vi "MenuSelection Response.vi"(6 "Coords":T1, 8 "error in (no error)":errorcluster, 9 "Menu Name":string, 10 "Menu Tag":string, 11 "UEF Handler1 in":refnum<class "UEF Handler2.lvclass">) -> (0 "error out":errorcluster, 3 "UEF Handler1 out":refnum<class "UEF Handler2.lvclass">)   [LabVIEW 2015, in "UEF Handler2.lvclass"]
uses:
  UEF Handler2.lvclass
  <vilib>/Utility/miscctls.llb/LVPoint32TypeDef.ctl
  <vilib>/LIEF/Forms/Rectangle/Rectangle.lvclass
  <vilib>/LIEF/Image Editor Handler/Image Editor Handler.lvclass/Image Editor Handler.ctl
  UEF Handler2.lvclass/UEF Handler2.ctl
  <vilib>/LIEF/Forms/Shape/Shape.lvclass/Shape.ctl
  <vilib>/LIEF/Forms/Rectangle/Rectangle.lvclass/Rectangle.ctl
  <vilib>/LIEF/Image Editor Handler/Read PictureRef.vi
  <vilib>/LIEF/Image Editor Handler/Read Shapes.vi
  <vilib>/LIEF/Forms/Shape/Write Color.vi
  <vilib>/LIEF/Forms/Rectangle/Write Filled.vi
  <vilib>/LIEF/Forms/Shape/Shape.lvclass
  <vilib>/LIEF/Image Editor Handler/Image Editor Handler.lvclass
  <vilib>/LIEF/Forms/Link/Link.lvclass
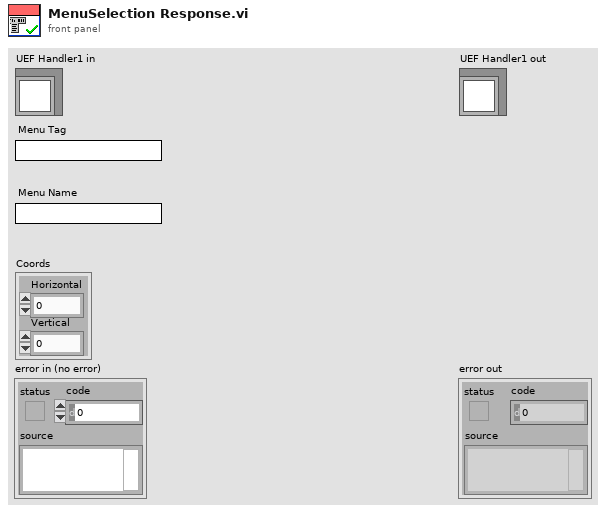
[diagram p1: front panel]
types:
  T1 = typedef "LVPoint32TypeDef.ctl" = cluster{"Horizontal":i32, "Vertical":i32}
  T2 = typedef "LVPositionTypeDef.ctl" = cluster{"Left":i32, "Top":i32}
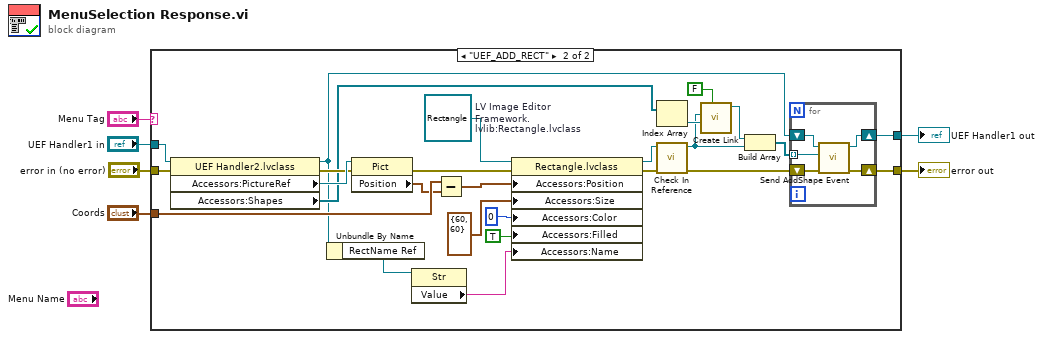
[diagram p0: block diagram]
diagram:
  n1 = case shown="\"UEF_ADD_RECT\"" "Menu Tag" {
    tunnel: "UEF Handler1 in" -> [w8 w34]
    tunnel: "Coords" -> [_ w32]
    tunnel: [w7 w23] -> w3
    tunnel: [w8 w22] -> w2
    tunnel: "error in (no error)" -> [w7 w18]
    frame "False", Default {
    }
    frame "UEF_ADD_RECT" {
      w30 = refnum<class "Rectangle.lvclass"> refnum  # LV Image Editor Framework.lvlib:Rectangle.lvclass
      n2 = property class="UEF Handler2.lvclass"(reference=w34, error in=w18) -> (reference out=w11:refnum<class "UEF Handler2.lvclass">, error out=w19:errorcluster, "Accessors:PictureRef"=w33:refnum<vi>, "Accessors:Shapes"=w17:refnum<data-value>[])
      n3 = Unbundle By Name(w11) -> ("RectName Ref"=w10:refnum<vi>)
      n4 = property class="Pict"(reference=w33, error in=w19) -> (error out=w20:errorcluster, "Position"=w31:T2)  [unwired: 1 out]
      n5 = property class="Str"(reference=w10) -> ("Value"=w9:string)  [unwired: 1 in, 2 out]
      n6 = Subtract(x=w32, y=w31) -> (x-y=w27:T1)
      n7 = property class="Rectangle.lvclass"(reference=w30, error in=w20, "Accessors:Position"=w27, "Accessors:Size"=cluster{"Width":i32, "Height":i32} {"Width"=60, "Height"=60} ("Size"), "Accessors:Color"=u32 0 ("Color"), "Accessors:Filled"=TRUE ("Filled"), "Accessors:Name"=w9) -> (reference out=w25:refnum<class "Rectangle.lvclass">, error out=w21:errorcluster)
      n8 = Index Array(array=w17) -> (element=w16:refnum<data-value>)  [unwired: 1 in]
      n9 = call <vilib>:"Check In Reference.vi"("error in (no error)"=w21, "Shape in"=w25) -> ("error out"=w24:errorcluster, "Shape Reference"=w14:refnum<data-value>)  [unwired: 8 in]
      n10 = call <vilib>:"Create Link.vi"("Selectable"=FALSE, "Destination"=w16, "Source"=w14) -> ("Link Reference"=w15:refnum<data-value>)  [unwired: 7 in, 1 out]
      n11 = Build Array(w15, w14) -> (w13:refnum<data-value>[])
      n12 = for {
        shift-right: [w36] -> w22
        shift-left: w11 -> [w39]
        shift-right: [w37] -> w23
        shift-left: w24 -> [w38]
        tunnel: w13 -> [w35] mode=indexing
        n13 = call <vilib>:"Send AddShape Event.vi"("error in (no error)"=w38, "New Shape Reference"=w35, "Editor Handler in"=w39) -> ("error out"=w37:errorcluster, "Editor Handler out"=w36:refnum<class "UEF Handler2.lvclass">)  [unwired: 7 in]
      }
    }
  }
  "error out" <- w3
  "UEF Handler1 out" <- w2
